vi "Temperature Monitor.vi"() -> ()   [LabVIEW 2019]
doc: "该VI是LabVIEW核心课程1中练习的答案。\n\n该VI使用While循环和移位寄存器进行均值计算。无需硬件。"
panel:
  in  "停止按钮":bool
  out "温度历史":cluster{dbl, "温度值":dbl}(graph)
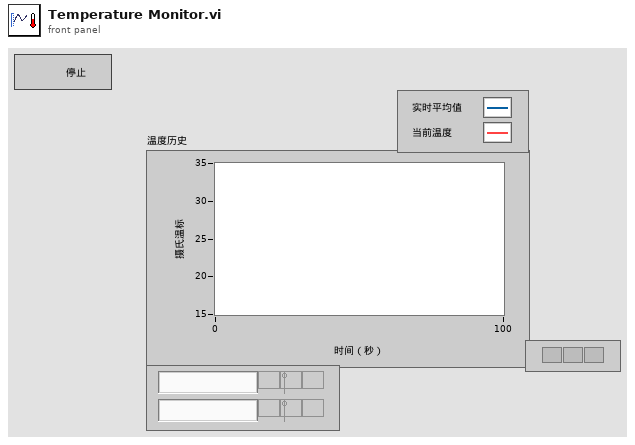
[diagram p1: front panel]
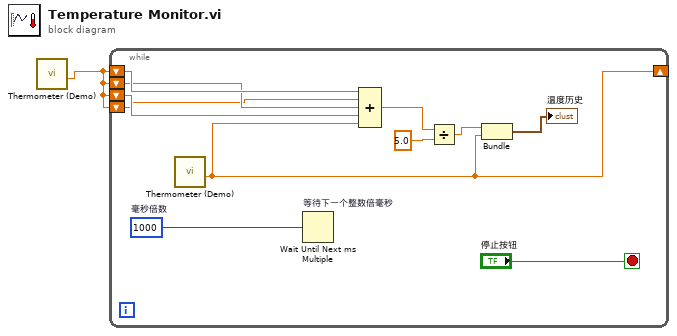
[diagram p0: block diagram]
diagram:
  n1 = call "Thermometer (Demo).vi"() -> ("温度值"=w1:dbl)  [unwired: 11 in]
  n2 = while {
    shift-right: [w3] -> _
    shift-left: w1 -> [w7]
    shift-left: w1 -> [w8]
    shift-left: w1 -> [w9]
    shift-left: w1 -> [w10]
    stop <- "停止按钮" stop-if-true
    w12 = u32 1000  # 毫秒倍数
    n3 = call "Thermometer (Demo).vi"() -> ("温度值"=w3:dbl)  [unwired: 11 in]
    n4 = Wait Until Next ms Multiple "等待下一个整数倍毫秒"(millisecond multiple=w12) -> ()  [unwired: 1 out]
    n5 = Compound Arithmetic op=ADD(w10, w7, w9, w8, w3) -> (w6:dbl)
    n6 = Divide(x=w6, y=5.0) -> (x/y=w4:dbl)
    n7 = Bundle(w4, "温度值"=w3) -> (→"温度历史":cluster{dbl, "温度值":dbl})  [unwired: 1 in]
  }
